vi "Init I2C_0-20mA(GP8313).vi"(8 "error in (no error)":errorcluster, 11 "I2C_0-20mA(GP8212) in":refnum<class "I2C_0-20mA(GP8313).lvclass">) -> (0 "error out":errorcluster, 3 "I2C_0-20mA(GP8212) out":refnum<class "I2C_0-20mA(GP8313).lvclass">)   [LabVIEW 2020, in "CTI-Peripheral.lvlib" / "I2C_0-20mA(GP8313).lvclass"]
uses:
  I2C_0-20mA(GP8313).lvclass
  I2C_0-20mA(GP8313).lvclass/I2C_0-20mA(GP8313).ctl
  CTI/I2C Connection/I2C Connection.lvclass/I2C Connection.ctl
  CTI/Session/I2C Write Data.vi
  CTI/I2C Connection/I2C Connection.lvclass
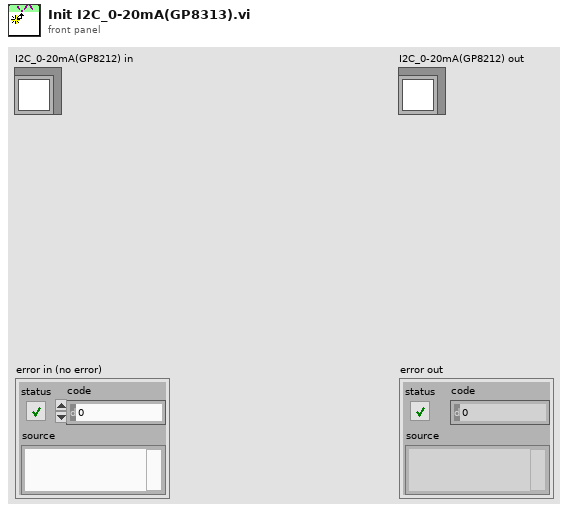
[diagram p1: front panel]
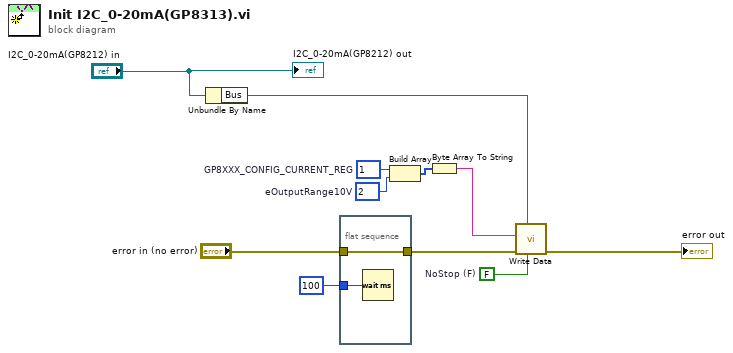
[diagram p0: block diagram]
diagram:
  w4 = u8 2  # eOutputRange10V
  w6 = u8 1  # GP8XXX_CONFIG_CURRENT_REG
  w9 = FALSE  # NoStop (F)
  n1 = Unbundle By Name("I2C_0-20mA(GP8212) in") -> ("Bus"=w10:refnum<class "I2C Connection.lvclass">)
  n2 = flat-sequence {
    tunnel: "error in (no error)" -> [w13]
    tunnel: [w13] -> w8
    tunnel: u32 100 ("milliseconds to wait") -> [w12]
    frame #0 {
      n3 = Wait (ms)(milliseconds to wait=w12) -> ()  [unwired: 1 out]
    }
  }
  n4 = Build Array(w6, w4) -> (w5:u8[])
  n5 = Byte Array To String(unsigned byte array=w5) -> (string=w1:string)
  n6 = call "Write Data.vi"("NoStop (F)"=w9, "I2C Connection"=w10, "error in (no error)"=w8, "Data"=w1) -> ("error out"=→"error out":errorcluster)  [unwired: 7 in]
  "I2C_0-20mA(GP8212) out" <- "I2C_0-20mA(GP8212) in"
